vi "Load Config.vi"(6 "Constants":refnum<class "Sequence Constants.lvclass">, 8 "error in (no error)":refnum<class "MultiErrors.lvclass">, 10 "Config Element":refnum<class "Config Element.lvclass">, 11 "Numeric Command Config in":refnum<class "Numeric Command Config.lvclass">) -> (0 "error out":refnum<class "MultiErrors.lvclass">, 3 "Numeric Command Config out":refnum<class "Numeric Command Config.lvclass">)   [LabVIEW 2020, in "VolatusSeqConfig.lvlib" / "Numeric Command Config.lvclass"]
uses:
  Numeric Command Config.lvclass
  VolatusErrorUtilities/MultiErrors/MultiErrors.lvclass
  lv-cdm/CDM-Config/Config Element/Config Element.lvclass
  Numeric Command Config.lvclass/Numeric Command Config.ctl
  Sequence Constants/Sequence Constants.lvclass
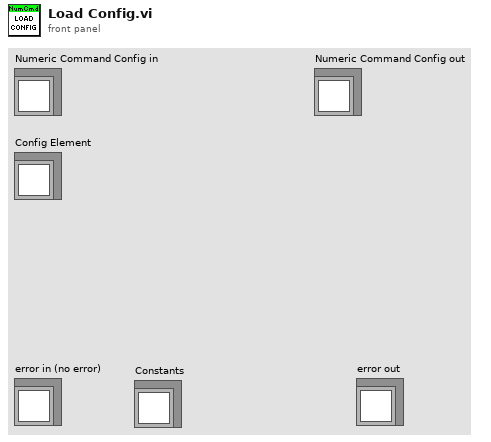
[diagram p1: front panel]
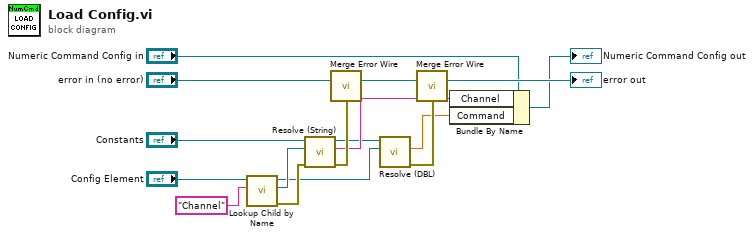
[diagram p0: block diagram]
diagram:
  n1 = call "Lookup Child by Name.vi"("Name"="Channel", "Config Element in"="Config Element") -> ("error out"=w7:errorcluster, "Child"=w6:refnum<class "Config Element.lvclass">, "Config Element out"=w3:refnum<class "Config Element.lvclass">)  [unwired: 6 in, 1 out]
  n2 = call "Resolve (String).vi"("error in (no error)"=w7, "Element"=w6, "Sequence Constants in"="Constants") -> ("error out"=w8:errorcluster, "String Value"=w5:string, "Sequence Constants out"=w4:refnum<class "Sequence Constants.lvclass">)  [unwired: 6 in]
  n3 = call "Merge Error Wire.vi"("error in (no error)"=w8, "MultiErrors in"="error in (no error)") -> ("MultiErrors out"=w10:refnum<class "MultiErrors.lvclass">)  [unwired: 13 in]
  n4 = call "Resolve (DBL).vi"("Element"=w3, "Sequence Constants in"=w4) -> ("error out"=w2:errorcluster, "DBL Value"=w1:dbl)  [unwired: 7 in, 1 out]
  n5 = call "Merge Error Wire.vi"("error in (no error)"=w2, "MultiErrors in"=w10) -> ("MultiErrors out"=→"error out":refnum<class "MultiErrors.lvclass">)  [unwired: 13 in]
  n6 = Bundle By Name(cluster="Numeric Command Config in", "Channel"=w5, "Command"=w1) -> (→"Numeric Command Config out":refnum<class "Numeric Command Config.lvclass">)
